vi "routine3.vi"(4 "amp3":dbl, 6 "amp1":dbl, 7 "section":i16, 11 "theta":dbl) -> (3 "x_d3":dbl)   [LabVIEW 2013]
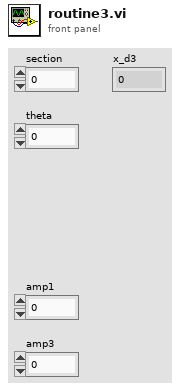
[diagram p1: front panel]
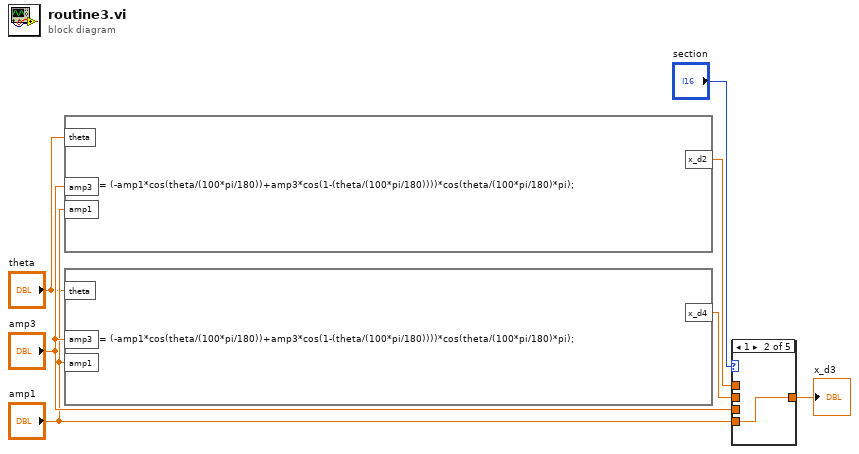
[diagram p0: block diagram]
diagram:
  n1 = formula code="x_d2 = (-amp1*cos(theta/(100*pi/180))+amp3*cos(1-(theta/(100*pi/180))))*cos(theta/(100*pi/180)*pi);"("theta"="theta", "amp3"="amp3", "amp1"="amp1") -> ("x_d2"=w5:dbl)
  n2 = formula code="x_d4 = (-amp1*cos(theta/(100*pi/180))+amp3*cos(1-(theta/(100*pi/180))))*cos(theta/(100*pi/180)*pi);"("theta"="theta", "amp3"="amp3", "amp1"="amp1") -> ("x_d4"=w7:dbl)
  n3 = case shown="1" "section" {
    tunnel: "amp1" -> [_ w8 _ _ _]
    tunnel: [_ w8 w9 w10 w11] -> w4
    tunnel: w5 -> [_ _ w9 _ _]
    tunnel: "amp3" -> [_ _ _ w10 _]
    tunnel: w7 -> [_ _ _ _ w11]
    frame 0, Default {
    }
    frame 1 {
    }
    frame 2 {
    }
    frame 3 {
    }
    frame 4 {
    }
  }
  "x_d3" <- w4
